vi "Deadzone.vi"(0 "Y":dbl, 3 "Deadzone":dbl=0.15 format="%#_13g") -> (9 "y with deadzone":dbl)   [LabVIEW 2013]
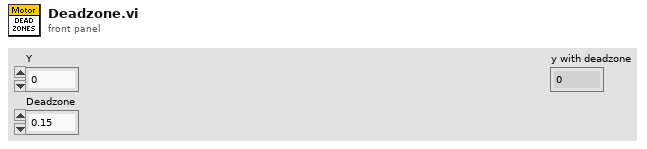
[diagram p1: front panel]
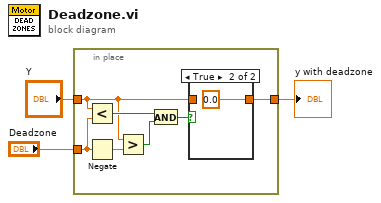
[diagram p0: block diagram]
diagram:
  n1 = in-place {
    in-place-border: "Y" -> [w7]
    in-place-border: [w6] -> w3
    in-place-border: "Deadzone" -> [w4]
    n2 = Less?(x=w7, y=w4) -> (x < y?=w10:bool)
    n3 = Negate(x=w4) -> (-x=w5:dbl)
    n4 = Greater?(x=w7, y=w5) -> (0:w9:bool)
    n5 = And(x=w10, y=w9) -> (x .and. y?=w8:bool)
    n6 = case shown="True" w8 {
      tunnel: w7 -> [w11 _]
      tunnel: [w11 0.0 ("Y")] -> w6
      frame False {
      }
      frame True {
      }
    }
  }
  "y with deadzone" <- w3
